vi "SetKparAxisMin.vi"(8 "error in (no error)":errorcluster, 9 "newMin":dbl, 10 "kPar":i32, 11 "dvotAFTKinetics in":refnum<class "dvotAFTKinetics.lvclass">) -> (0 "error out":errorcluster, 3 "dvotAFTKinetics out":refnum<class "dvotAFTKinetics.lvclass">)   [LabVIEW 2012, in "dvotAFTKinetics.lvclass"]
uses:
  dvotAFTKinetics.lvclass
  dvotAFTKinetics.lvclass/dvotAFTKinetics.ctl
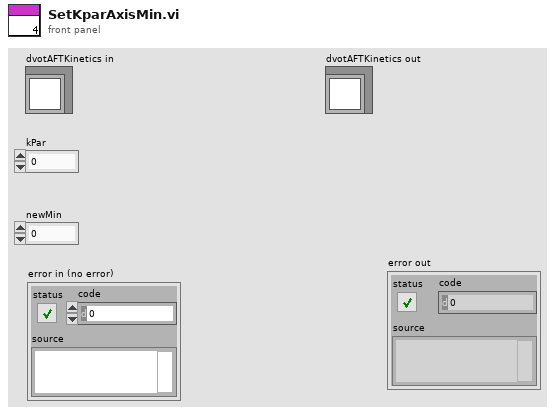
[diagram p1: front panel]
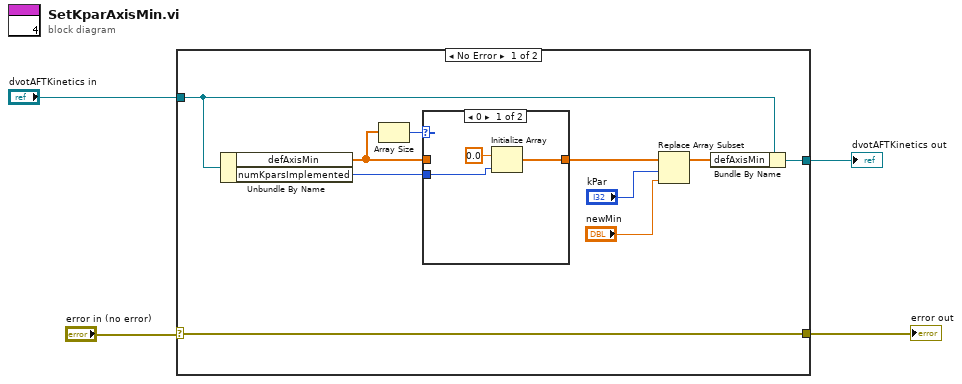
[diagram p0: block diagram]
diagram:
  n1 = case shown="No Error" "error in (no error)" {
    selector: "error in (no error)" -> [w11 w19]
    tunnel: "dvotAFTKinetics in" -> [w14 w20]
    tunnel: [w12 w20] -> w1
    tunnel: [w11 w19] -> w4
    frame No Error {
      n2 = Unbundle By Name(w14) -> ("defAxisMin"=w9:dbl[], "numKparsImplemented"=w7:i32)
      n3 = Array Size(array=w9) -> (size(s)=w10:i32)
      n4 = case shown="0" w10 {
        tunnel: w9 -> [_ w18]
        tunnel: [w17 w18] -> w8
        tunnel: w7 -> [w15 _]
        frame 0 {
          n5 = Initialize Array(0.0 ("element"), w15) -> (w17:dbl[])
        }
        frame Default {
        }
      }
      n6 = Replace Array Subset(array=w8, new element="newMin", index="kPar") -> (w13:dbl[])
      n7 = Bundle By Name(cluster=w14, "defAxisMin"=w13) -> (w12:refnum<class "dvotAFTKinetics.lvclass">)
    }
    frame Error {
    }
  }
  "error out" <- w4
  "dvotAFTKinetics out" <- w1
